vi "Configure_Interrupts.vi"(7 "I2C Channel":u8, 8 "error in":errorcluster, 10 "Interrupts Settings":T1={"Interrupt Level"=48, "Interrupt Pad Mode"=48, "<INT2_SRC> Latch Request"=48, "Data Signal on INT2 Pad"=48, "<INT1_SRC> Latch Request"=48, "Data Signal on INT1 Pad"=48} {"Data Signal on INT1 Pad" items=["Interrupt 1 Source", "Int. 1 Source OR Int. 2 Source", "Data Ready", "Boot Running"]; "<INT1_SRC> Latch Request" items=["Interrupt Request Not Latched"=0, "Interrupt Request Latched"=4]; "Data Signal on INT2 Pad" items=["Interrupt 2 Source"=0, "Int. 1 Source OR Int. 2 Source"=8, "Data Ready"=16, "Boot Running"=24]; "<INT2_SRC> Latch Request" items=["Interrupt Request Latched"=32, "Interrupt Request Not Latched"=0]; "Interrupt Pad Mode" items=["Open-Drain"=64, "Push-Pull"=0]; "Interrupt Level" items=["Interrupt Active LOW"=128, "Interrupt Active HIGH"=0]}, 11 "LINX Resource In":T2) -> (0 "error out":errorcluster, 3 "LINX Resource Out":T2)   [LabVIEW 2014, in "LMH-LINX.lvlib" / "LIS331HH.lvlib"]
uses:
  <vilib>/MakerHub/LINX/Public/Sensors/Accelerometer/LIS331HH/LIS331HH.lvlib
  <vilib>/MakerHub/LINX/Private/Type Defs/LINX Ref.ctl
  <vilib>/MakerHub/LINX/Private/Type Defs/Platform.ctl
  <vilib>/MakerHub/LINX/Private/Type Defs/Interface.ctl
  <vilib>/MakerHub/LINX/Private/Device/Type Defs/LINX Device Config.ctl
  <vilib>/MakerHub/LINX/Private/Device/Type Defs/TCP Config.ctl
  <vilib>/MakerHub/LINX/Private/Device/Type Defs/Channels.ctl
  <vilib>/MakerHub/LINX/Public/Sensors/Accelerometer/LIS331HH/Controls/CTRL_REG3.ctl
  <vilib>/MakerHub/LINX/Private/Local IO/LinxI2cWrite.vi
  <vilib>/MakerHub/LINX/Public/Utilities/Check Channel.vi
  <vilib>/MakerHub/LINX/Private/Utilties/Generate Error.vi
  <vilib>/MakerHub/LINX/LMH-LINX.lvlib
  <vilib>/MakerHub/LINX/Private/Device/Device.lvlib
panel:
  # "OUTPUTS"
  # "INPUTS"
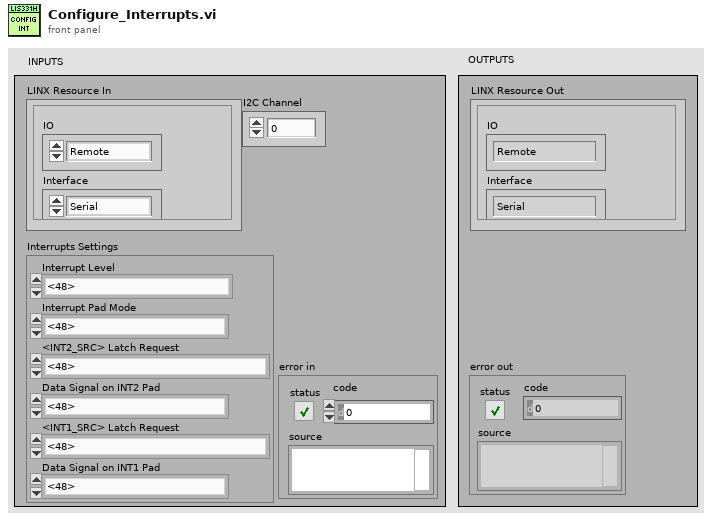
[diagram p1: front panel]
types:
  T1 = typedef "LMH-LINX.lvlib/LIS331HH.lvlib/CTRL_REG3.ctl" = cluster{"Interrupt Level":u8, "Interrupt Pad Mode":u8, "<INT2_SRC> Latch Request":u8, "Data Signal on INT2 Pad":u8, "<INT1_SRC> Latch Request":u8, "Data Signal on INT1 Pad":u8}
  T2 = typedef "LMH-LINX.lvlib/LINX Ref.ctl" = cluster{"IO":T3, "Interface":T4, "LINX Device Config":T5}
  T3 = typedef "LMH-LINX.lvlib/Platform.ctl" = enum16{"Remote", "Local"}
  T4 = typedef "LMH-LINX.lvlib/Interface.ctl" = enum16{"Serial", "TCP"}
  T5 = typedef "LMH-LINX.lvlib/Device.lvlib/LINX Device Config.ctl" = cluster{"Interface":T4, "COM Port":refnum<visa-resource-name>, "TCP Configuration":T6, "Device Family":u8, "Device ID":u8, "Device Name":string, "TCP Ref":refnum<k5>, "Channels":T7}
  T6 = typedef "LMH-LINX.lvlib/Device.lvlib/TCP Config.ctl" = cluster{"IP Address":string, "Port":u16}
  T7 = typedef "LMH-LINX.lvlib/Channels.ctl" = cluster{"DI":u8[], "DO":u8[], "AI":u8[], "AO":u8[], "PWM":u8[], "QE":u8[], "UART":u8[], "I2C 2":u8[], "SPI":u8[], "CAN":u8[], "Servo":u8[], "AI Ref (V)":dbl, "AI Resolution (Bits)":u8, "AO Ref (V)":dbl, "AO Resolution (Bits)":u8}
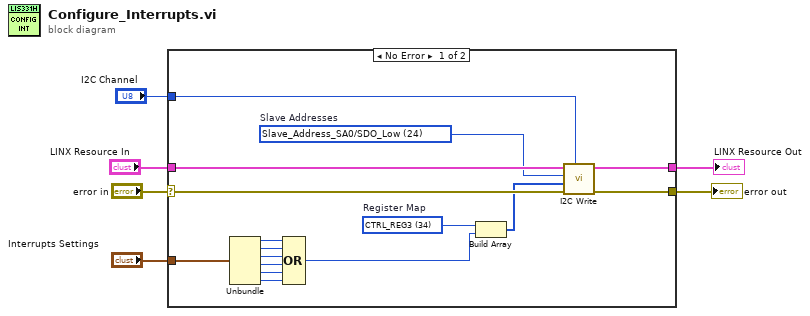
[diagram p0: block diagram]
diagram:
  n1 = case shown="No Error" "error in" {
    selector: "error in" -> [w21 w24]
    tunnel: [w17 w24] -> w5
    tunnel: "LINX Resource In" -> [w22 w23]
    tunnel: "I2C Channel" -> [w19 _]
    tunnel: [w18 w23] -> w2
    tunnel: "Interrupts Settings" -> [w14 _]
    frame No Error {
      w15 = u8 24 items=["Slave_Address_SA0/SDO_Low"=24, "Slave_Address_SA0/SDO_High"=25]  # Slave Addresses
      w16 = u8 34 items=["CTRL_REG1"=32, "CTRL_REG2"=33, "CTRL_REG3"=34, "CTRL_REG4"=35, "CTRL_REG5"=36, "HP_FILTER_RESET"=37, "REFERENCE"=38, "STATUS_REG"=39, "OUT_X_L"=40, "OUT_X_H"=41, "OUT_Y_L"=42, "OUT_Y_H"=43, "OUT_Z_L"=44, "OUT_Z_H"=45, "INT1_CFG"=48, "INT1_SOURCE"=49, "INT1_THS"=50, "INT1_DURATION"=51, "INT2_CFG"=52, "INT2_SOURCE"=53, "INT2_THS"=54, "INT2_DURATION"=55]  # Register Map
      n2 = Unbundle(w14) -> ("Interrupt Level"=w13:u8, "Interrupt Pad Mode"=w12:u8, "<INT2_SRC> Latch Request"=w11:u8, "Data Signal on INT2 Pad"=w10:u8, "<INT1_SRC> Latch Request"=w8:u8, "Data Signal on INT1 Pad"=w7:u8)
      n3 = Compound Arithmetic op=OR(w13, w12, w11, w10, w8, w7) -> (w9:u8)
      n4 = Build Array(w16, w9) -> (w20:u8[])
      n5 = call <vilib>:"I2C Write.vi"("I2C Channel"=w19, "Error In"=w21, "Data"=w20, "I2C Slave Address (0)"=w15, "LINX Resource"=w22) -> ("Error Out"=w17:errorcluster, "LINX Resource"=w18:T2)  [unwired: 5 in]
    }
    frame Error {
    }
  }
  "error out" <- w5
  "LINX Resource Out" <- w2
